vi "IOTdata操作函数.vi"(9 "IOTdata集合输入":T1, 11 "操作选项":enum16{"初始化", "获取参数", "写入参数"}(ring)) -> (3 "IOTdata集合":T1)   [LabVIEW 2017]
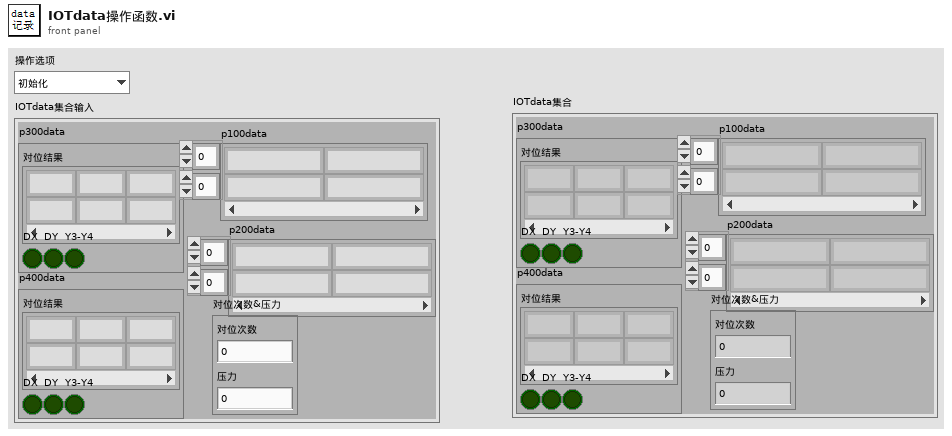
[diagram p1: front panel]
types:
  T1 = typedef "IOTdata集合.ctl" = cluster{"p300data":T2, "p400data":T2, "p100data":string[][], "p200data":string[][], "对位次数&压力":cluster{"对位次数":dbl, "压力":dbl}}
  T2 = typedef "P300&P400结果.ctl" = cluster{"对位结果":string[][], "DX":bool, "DY":bool, "Y3-Y4":bool}
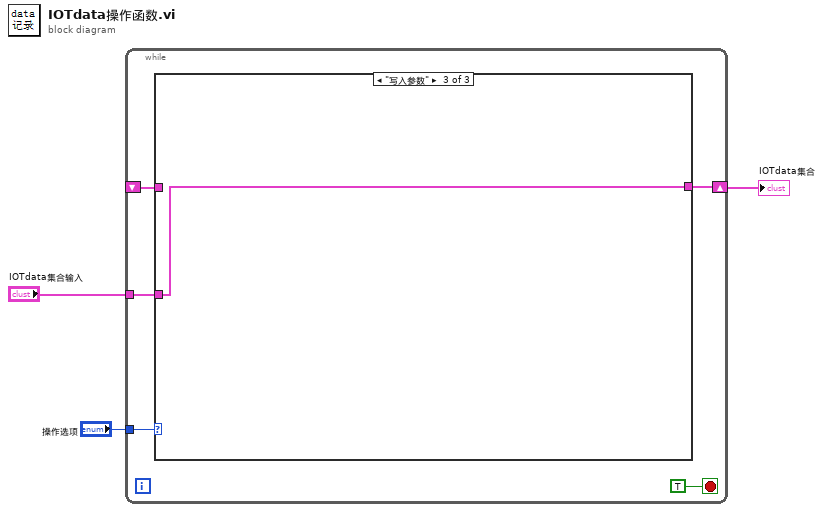
[diagram p0: block diagram]
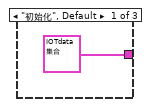
[diagram p2: hidden frame]
diagram:
  n1 = while {
    tunnel: "操作选项" -> [w7]
    shift-right: [w5] -> w2
    shift-left: _ -> [w4]
    tunnel: "IOTdata集合输入" -> [w6]
    stop <- TRUE stop-if-true
    n2 = case shown="\"写入参数\"" w7 {
      tunnel: w6 -> [_ _ w11]
      tunnel: [T1 {"p300data"={"对位结果"=[], "DX"=FALSE, "DY"=FALSE, "Y3-Y4"=FALSE}, "p400data"={"对位结果"=[], "DX"=FALSE, "DY"=FALSE, "Y3-Y4"=FALSE}, "p100data"=[], "p200data"=[], "对位次数&压力"={"对位次数"=0.0, "压力"=0.0}} ("IOTdata集合") w10 w11] -> w5
      tunnel: w4 -> [_ w10 _]
      frame "初始化", Default {
      }
      frame "获取参数" {
      }
      frame "写入参数" {
      }
    }
  }
  "IOTdata集合" <- w2
